vi "_Get UI Details.vi"(8 "error in (no error)":errorcluster) -> (0 "error out":errorcluster, 3 "user interface details":T1[](array[typedef]))   [LabVIEW 2021, in "MeasurementServerTests.lvlib" / "Measurement Service Tests.lvlib" / "Continuous Counting Measurement.lvclass"]
uses:
  Continuous Counting Measurement.lvclass
  Runtime/Measurements/Helpers/TypeDefs/User Interface Information.ctl
  Runtime/Measurements/NI Measurement Plug-In SDK.lvlib
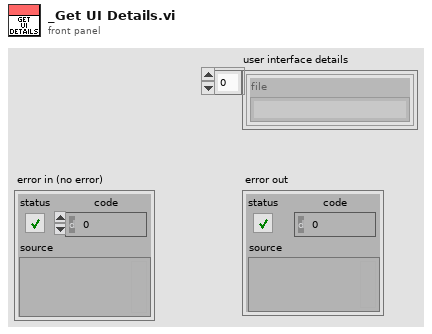
[diagram p1: front panel]
types:
  T1 = typedef "NI Measurement Plug-In SDK.lvlib/User Interface Information.ctl" = cluster{"file":string}
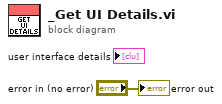
[diagram p0: block diagram]
diagram:
  "error out" <- "error in (no error)"
